vi "Actor Last Ack.vi"(9 "Nest Error":errorcluster, 10 "Nest Actor":refnum<class "Actor.lvclass">, 11 "Self Actor in":refnum<class "Self Actor.lvclass">) -> (0 "error out":errorcluster, 3 "Self Actor out":refnum<class "Self Actor.lvclass">)   [LabVIEW 2021, in "LVCAM.lvlib" / "Self Actor.lvclass"]
uses:
  Self Actor.lvclass
  Actor/Actor.lvclass
  Self Actor.lvclass/Self Actor.ctl
  LVCAM.lvlib
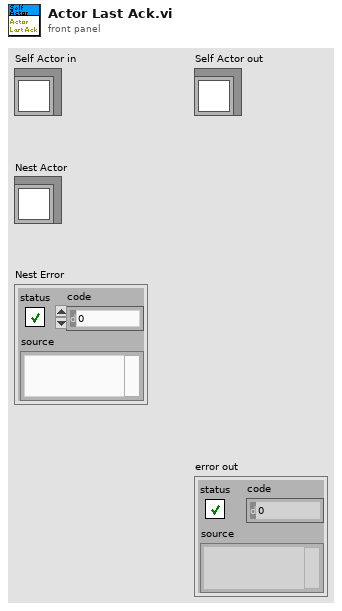
[diagram p1: front panel]
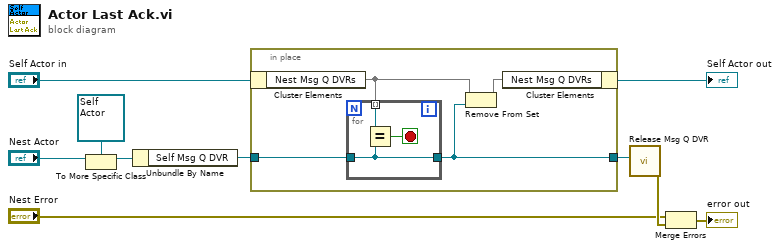
[diagram p0: block diagram]
diagram:
  n1 = To More Specific Class(target class=refnum<class "Self Actor.lvclass"> refnum ("Artifex Actor Model.lvlib:Self Actor.lvclass"), reference="Nest Actor") -> (specific class reference=w10:refnum<class "Self Actor.lvclass">)  [unwired: 1 in, 1 out]
  n2 = Unbundle By Name(w10) -> ("Self Msg Q DVR"=w6:refnum<data-value>)
  n3 = in-place {
    in-place-border: w6 -> [w12]
    in-place-border: [w11] -> w5
    n4 = in-place-cluster #1("Self Actor in") -> ("Nest Msg Q DVRs"=w14:set{refnum<data-value>})
    n5 = for {
      tunnel: w12 -> [w15]
      tunnel: w14 -> [w16] mode=indexing
      tunnel: [w15] -> w11
      stop <- w17 stop-if-true
      n6 = Equal?(x=w16, y=w15) -> (x = y?=w17:bool)
    }
    n7 = Remove From Set(10:w11, 11:w14) -> (3:w13:set{refnum<data-value>})  [unwired: 1 out]
    n8 = in-place-cluster #1("Nest Msg Q DVRs"=w13) -> (→"Self Actor out":refnum<class "Self Actor.lvclass">)
  }
  n9 = call "Release Msg Q DVR.vi"("Msg Q DVR"=w5) -> ("error out"=w3:errorcluster)  [unwired: 10 in]
  n10 = Merge Errors("Nest Error", w3) -> (→"error out":errorcluster)
